vi "ReadMultiPointLowLevel.vi"(4 "iTriggerCount":i32, 6 "iMaxTimeMilliseconds":u32=10000, 8 "error in (no error)":errorcluster, 9 "dSampleInterval":dbl format="%_4e", 10 "iArraySize":i32, 11 "Handle":refnum<visa-resource-name>) -> (0 "error out":errorcluster, 2 "iActualPts":i32, 3 "dReadingArray":dbl[](array[numeric]) caption="Muestras digitales" format="%^.3e")   [LabVIEW 2014, in "SamplerPlugins.lvlib" / "HP3458aDMM.lvclass"]
uses:
  HP3458aDMM.lvclass
  <instrlib>/Agilent 3458/Agilent 3458.lvlib
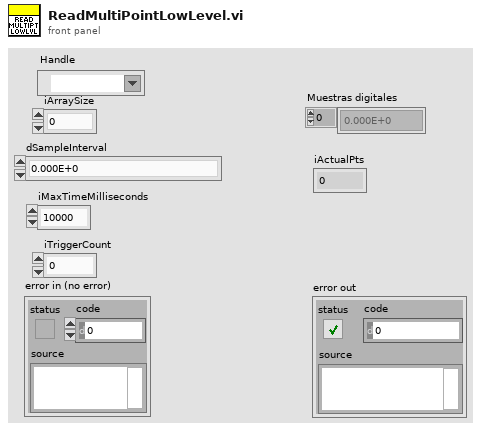
[diagram p1: front panel]
types:
  T1 = enum16{"ASCII", "Single Real", "Double Real", "Single Integer", "Double Integer"}
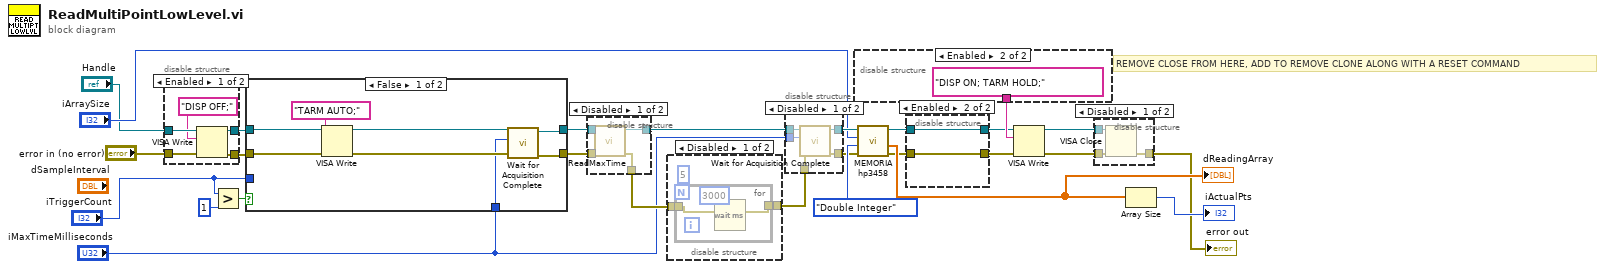
[diagram p0: block diagram]
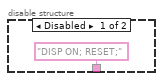
[diagram p4: hidden frame]
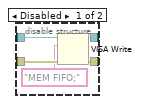
[diagram p7: hidden frame]
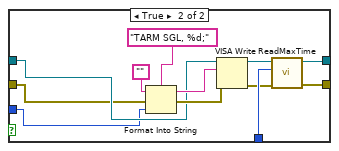
[diagram p9: hidden frame]
diagram:
  # "REMOVE CLOSE FROM HERE, ADD TO REMOVE CLONE ALONG WITH A RESET COMMAND"
  n1 = disable-structure shown="Enabled" {
    disable-tunnel: "error in (no error)" -> [w32 w33]
    disable-tunnel: [w31 w33] -> w3
    disable-tunnel: [w30 w34] -> w2
    disable-tunnel: "Handle" -> [w29 w34]
    frame Enabled {
      n2 = VISA Write(VISA resource name=w29, write buffer="DISP OFF;", error in (no error)=w32) -> (VISA resource name out=w30:refnum<visa-resource-name>, error out=w31:errorcluster)  [unwired: 1 out]
    }
    frame Disabled {
    }
  }
  n3 = Greater?(x="iTriggerCount", y=1) -> (0:w11:bool)
  n4 = case shown="False" w11 {
    tunnel: w2 -> [w41 w50]
    tunnel: w3 -> [w40 w49]
    tunnel: [w36 w44] -> w8
    tunnel: "iTriggerCount" -> [_ w48]
    tunnel: [w38 w43] -> w9
    tunnel: "iMaxTimeMilliseconds" -> [w35 w46]
    frame False {
      n5 = VISA Write(VISA resource name=w41, write buffer="TARM AUTO;", error in (no error)=w40) -> (VISA resource name out=w39:refnum<visa-resource-name>, error out=w37:errorcluster)  [unwired: 1 out]
      n6 = call <instrlib>:"Wait for Acquisition Complete.vi"("error in (no error)"=w37, "Maximum Time (10000 ms)"=w35, "VISA resource name"=w39) -> ("error out"=w36:errorcluster, "VISA resource name out"=w38:refnum<visa-resource-name>)  [unwired: 7 in]
    }
    frame True {
      n7 = Format Into String(format string="TARM SGL, %d;", initial string="", error in=w49, w48) -> (resulting string=w52:string, error out=w51:errorcluster)
      n8 = VISA Write(VISA resource name=w50, write buffer=w52, error in (no error)=w51) -> (VISA resource name out=w47:refnum<visa-resource-name>, error out=w45:errorcluster)  [unwired: 1 out]
      n9 = call "ReadMaxTime.vi"("error in (no error)"=w45, "iMaxTimeMilliseconds"=w46, "HandleIn"=w47) -> ("error out"=w44:errorcluster, "HandleOut"=w43:refnum<visa-resource-name>)  [unwired: 7 in]
    }
  }
  n10 = disable-structure shown="Disabled" {
    disable-tunnel: w9 -> [w58 w59]
    disable-tunnel: w8 -> [w57 w60]
    disable-tunnel: [w56 w59] -> w7
    disable-tunnel: [w55 w60] -> w6
    frame Disabled {
      n11 = call "ReadMaxTime.vi"("error in (no error)"=w57, "HandleIn"=w58) -> ("error out"=w55:errorcluster, "HandleOut"=w56:refnum<visa-resource-name>)  [unwired: 8 in]
    }
    frame Enabled {
    }
  }
  n12 = disable-structure shown="Disabled" {
    disable-tunnel: [w63 w66] -> w10
    disable-tunnel: w6 -> [w61 w66]
    frame Disabled {
      n13 = for {
        N: 5 -> [_]
        tunnel: [w65] -> w63
        tunnel: w61 -> [w65]
        n14 = Wait (ms)(milliseconds to wait=u32 3000) -> ()  [unwired: 1 out]
      }
    }
    frame Enabled {
    }
  }
  n15 = disable-structure shown="Disabled" {
    disable-tunnel: [w71 w72] -> w23
    disable-tunnel: [w70 w73] -> w22
    disable-tunnel: w10 -> [w69 w72]
    disable-tunnel: w7 -> [w68 w73]
    disable-tunnel: "iMaxTimeMilliseconds" -> [w67 _]
    frame Disabled {
      n16 = call <instrlib>:"Wait for Acquisition Complete.vi"("error in (no error)"=w69, "Maximum Time (10000 ms)"=w67, "VISA resource name"=w68) -> ("error out"=w71:errorcluster, "VISA resource name out"=w70:refnum<visa-resource-name>)  [unwired: 7 in]
    }
    frame Enabled {
    }
  }
  n17 = disable-structure shown="Enabled" {
    disable-tunnel: ["DISP ON; RESET;" ("write buffer") "DISP ON; TARM HOLD;" ("write buffer")] -> w20
    frame Disabled {
    }
    frame Enabled {
    }
  }
  n18 = call "MEMORIA hp3458.vi"("error in (no error)"=w23, "Output Format (0:ASCII)"=T1."Double Integer", "Número de muestras totales"="iArraySize", "VISA session"=w22) -> ("error out"=w24:errorcluster, "Muestras digitales"=w26:dbl[], "dup VISA session"=w25:refnum<visa-resource-name>)  [unwired: 4 in, 1 out]
  "dReadingArray" <- w26
  n19 = disable-structure shown="Enabled" {
    disable-tunnel: w25 -> [w80 w82]
    disable-tunnel: w24 -> [w79 w81]
    disable-tunnel: [w77 w82] -> w17
    disable-tunnel: [w76 w81] -> w16
    frame Disabled {
      n20 = VISA Write(VISA resource name=w80, write buffer="MEM FIFO;", error in (no error)=w79) -> (VISA resource name out=w77:refnum<visa-resource-name>, error out=w76:errorcluster)  [unwired: 1 out]
    }
    frame Enabled {
    }
  }
  n21 = VISA Write(VISA resource name=w17, write buffer=w20, error in (no error)=w16) -> (VISA resource name out=w19:refnum<visa-resource-name>, error out=w18:errorcluster)  [unwired: 1 out]
  n22 = disable-structure shown="Disabled" {
    disable-tunnel: w19 -> [w85 _]
    disable-tunnel: w18 -> [w84 w86]
    disable-tunnel: [w83 w86] -> w14
    frame Disabled {
      n23 = VISA Close(VISA resource name=w85, error in (no error)=w84) -> (error out=w83:errorcluster)
    }
    frame Enabled {
    }
  }
  "error out" <- w14
  n24 = Array Size(array=w26) -> (size(s)=→"iActualPts":i32)
